vi "FTW-Actor-LocalMessage-Send-Lossy.vi"(0 "FTW-ActorInstance In":refnum<class "FTW-ActorInstance.lvclass">, 5 "Message Header":string, 7 "Message Body":string, 11 "error in":errorcluster) -> (15 "error out":errorcluster)   [LabVIEW 2013, in "FTW-ActorInstance.lvclass"]
uses:
  FTW-ActorInstance.lvclass
  Message/Lossy/FTW-Message-Lossy.lvclass
  FTW-ActorInstance.lvclass/FTW-ActorInstance.ctl
  Message/Base/FTW-Message.lvclass
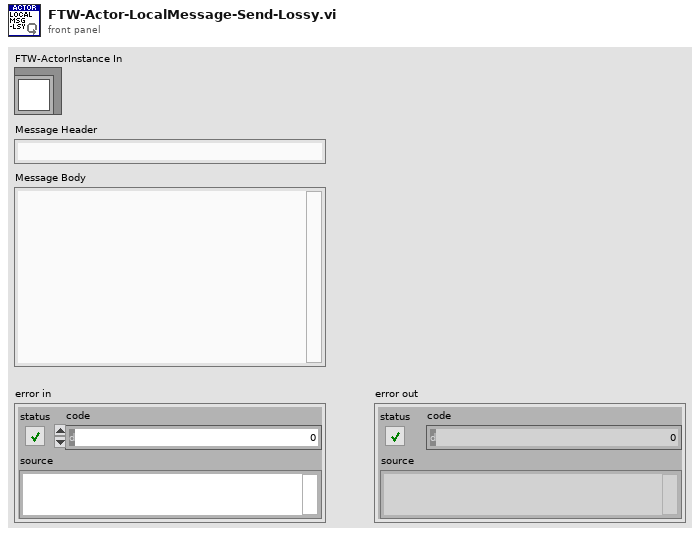
[diagram p1: front panel]
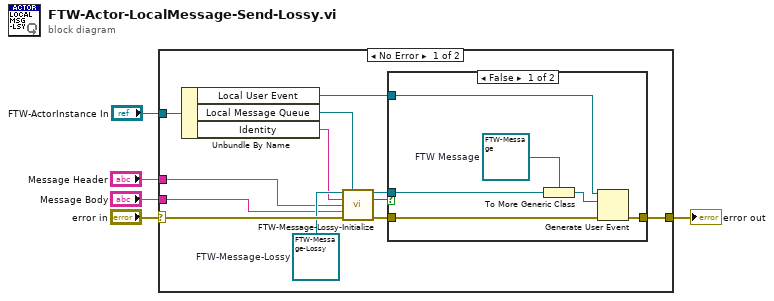
[diagram p0: block diagram]
diagram:
  n1 = case shown="No Error" "error in" {
    selector: "error in" -> [w14 w25]
    tunnel: "FTW-ActorInstance In" -> [w15 _]
    tunnel: [w13 w25] -> w3
    tunnel: "Message Header" -> [w8 _]
    tunnel: "Message Body" -> [w7 _]
    frame No Error {
      w12 = refnum<class "FTW-Message-Lossy.lvclass"> refnum  # FTW-Message-Lossy
      n2 = Unbundle By Name(w15) -> ("Local User Event"=w11:refnum<user-event>, "Local Message Queue"=w10:refnum<queue>, "Identity"=w9:string)
      n3 = call-dynamic "FTW-Message-Lossy-Initialize.vi"("FTW-Message-Lossy In"=w12, "Queue"=w10, "Sender Identity"=w9, "Message Header"=w8, "Message Body"=w7, "error in"=w14) -> ("FTW-Message-Lossy Out"=w16:refnum<class "FTW-Message-Lossy.lvclass">, "overflow?"=w6:bool, "error out"=w17:errorcluster)  [unwired: 7 in]
      n4 = case shown="False" w6 {
        tunnel: w17 -> [w22 w24]
        tunnel: w16 -> [w21 _]
        tunnel: [w20 w24] -> w13
        tunnel: w11 -> [w18 _]
        frame False {
          w19 = refnum<class "FTW-Message.lvclass"> refnum  # FTW Message
          n5 = To More Generic Class(target class=w19, reference=w21) -> (generic class reference=w23:refnum<class "FTW-Message.lvclass">)
          n6 = Generate User Event(user event=w18, event data cluster=w23, error in=w22) -> (error out=w20:errorcluster)  [unwired: 1 in, 1 out]
        }
        frame True {
        }
      }
    }
    frame Error {
    }
  }
  "error out" <- w3
